vi "accurus_button_control.vi"(11 "Array in":bool[](array[boolean])) -> (3 "Array out":bool[](array[boolean]))   [LabVIEW 2016]
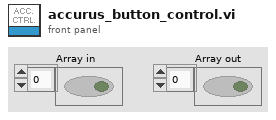
[diagram p1: front panel]
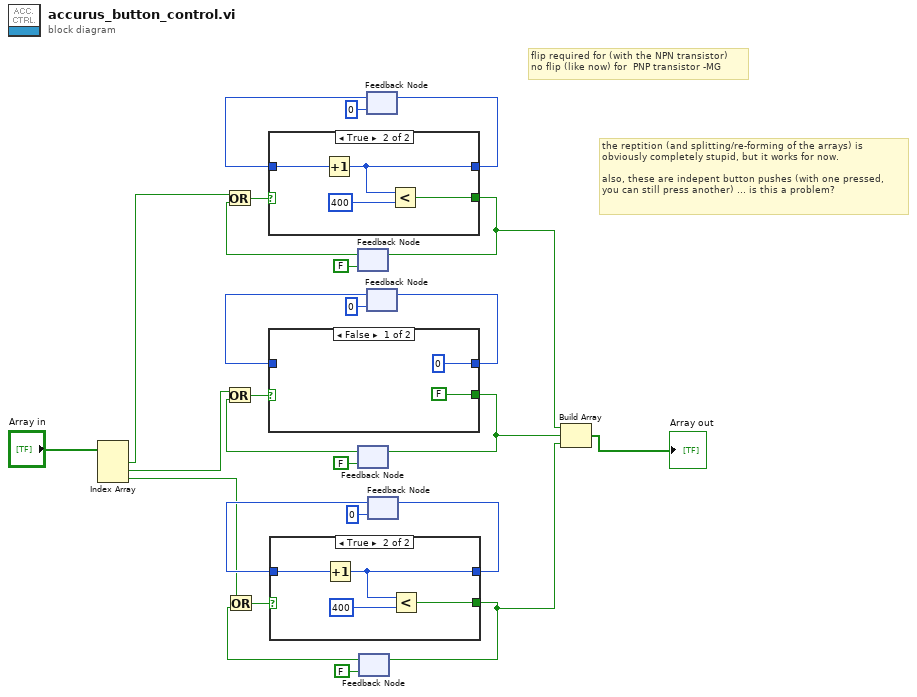
[diagram p0: block diagram]
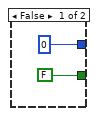
[diagram p2: hidden frame]
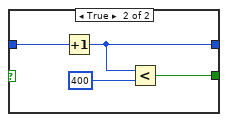
[diagram p3: hidden frame]
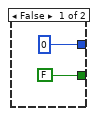
[diagram p4: hidden frame]
diagram:
  # "flip required for (with the NPN transistor)\nno flip (like now) for  PNP transistor -MG"
  # "the reptition (and splitting/re-forming of the arrays) is \nobviously completely stupid, but it works for now. \n\nalso, these are indepent button pushes (with one pressed, \nyou can still press another) ... is this a problem?"
  n1 = Index Array(array="Array in") -> (element #1=w26:bool, element #2=w5:bool, element #3=w6:bool)  [unwired: 3 in]
  n2 = feedback #1(FALSE) -> (w24:bool)
  n3 = Or(x=w26, y=w24) -> (x .or. y?=w23:bool)
  n4 = feedback #2(FALSE) -> (w18:bool)
  n5 = Or(x=w5, y=w18) -> (x .or. y?=w17:bool)
  n6 = feedback #3(FALSE) -> (w12:bool)
  n7 = Or(x=w6, y=w12) -> (x .or. y?=w11:bool)
  n8 = feedback #4(0) -> (w20:i32)
  n9 = case shown="True" w23 {
    tunnel: [0 w30] -> w19
    tunnel: w20 -> [_ w32]
    tunnel: [FALSE w29] -> w2
    frame False {
    }
    frame True {
      n10 = Increment(x=w32) -> (x+1=w30:i32)
      n11 = Less?(x=w30, y=400) -> (x < y?=w29:bool)
    }
  }
  n12 = feedback-in #1(w2) -> ()
  n13 = feedback-in #4(w19) -> ()
  n14 = feedback #5(0) -> (w14:i32)
  n15 = case shown="False" w17 {
    tunnel: [0 w36] -> w13
    tunnel: w14 -> [_ w38]
    tunnel: [FALSE w35] -> w3
    frame False {
    }
    frame True {
      n16 = Increment(x=w38) -> (x+1=w36:i32)
      n17 = Less?(x=w36, y=400) -> (x < y?=w35:bool)
    }
  }
  n18 = feedback-in #2(w3) -> ()
  n19 = feedback-in #5(w13) -> ()
  n20 = feedback #6(0) -> (w8:i32)
  n21 = case shown="True" w11 {
    tunnel: [0 w42] -> w7
    tunnel: w8 -> [_ w44]
    tunnel: [FALSE w41] -> w4
    frame False {
    }
    frame True {
      n22 = Increment(x=w44) -> (x+1=w42:i32)
      n23 = Less?(x=w42, y=400) -> (x < y?=w41:bool)
    }
  }
  n24 = feedback-in #3(w4) -> ()
  n25 = feedback-in #6(w7) -> ()
  n26 = Build Array(w2, w3, w4) -> (→"Array out":bool[])
